vi "Reporting_error.vi"(1 "error out 2":errorcluster, 2 "Concept explanation":string, 3 "Concept":string) -> (0 "Reporting":string)   [LabVIEW 2015]
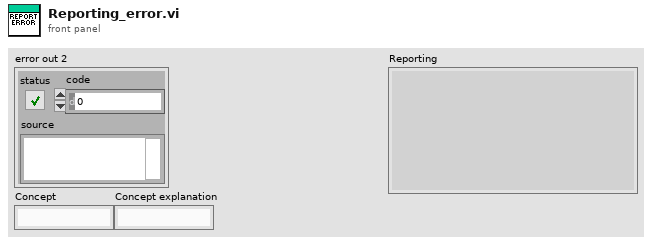
[diagram p1: front panel]
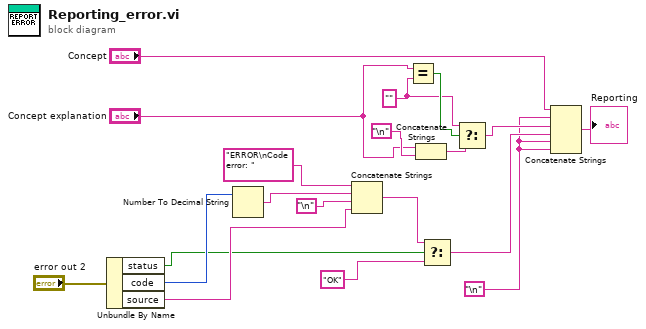
[diagram p0: block diagram]
diagram:
  w2 = "\n"
  w4 = ""
  n1 = Unbundle By Name("error out 2") -> ("status"=w1:bool, "code"=w18:i32, "source"=w7:string)
  n2 = Number To Decimal String(number=w18) -> (decimal integer string=w16:string)  [unwired: 1 in]
  n3 = Concatenate Strings("ERROR\nCode error: ", w16, "\n", w7) -> (w14:string)
  n4 = Equal?(x="Concept explanation", y=w4) -> (x = y?=w13:bool)
  n5 = Concatenate Strings("Concept explanation", "\n") -> (w5:string)
  n6 = Select(t=w14, s=w1, f="OK") -> (s? t:f=w10:string)
  n7 = Select(t=w4, s=w13, f=w5) -> (s? t:f=w11:string)
  n8 = Concatenate Strings("Concept", w2, w11, w10, w2, w2) -> (→"Reporting":string)
